vi "Register gRPC Methods.vi"(8 "error in (no error)":errorcluster, 11 "Template Server in":refnum<class "ctet_smu.lvclass">) -> (0 "error out":errorcluster, 3 "Template Server out":refnum<class "ctet_smu.lvclass">)   [LabVIEW 2019, in "ctet_smu.lvlib" / "ctet_smu.lvclass"]
uses:
  ctet_smu.lvclass
  typeDefs/Server Internal UEs.ctl
  typeDefs/Server Internal Message.ctl
  typeDefs/Server gRPC UEs.ctl
  gRPC lvSupport/Server API/typeDefs/gRPCId Cluster.ctl
  gRPC lvSupport/Server API/typeDefs/grpcId.ctl
  ctet_smu.lvclass/ctet_smu.ctl
  gRPC lvSupport/gprc-lvsupport.lvlib
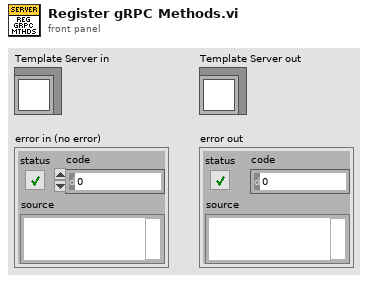
[diagram p1: front panel]
types:
  T1 = typedef "ctet_smu.lvlib/ctet_smu.lvclass/Server gRPC UEs.ctl" = cluster{"Invoke gRPC UE":refnum<user-event>, "Query gRPC UE":refnum<user-event>, "Register gRPC UE":refnum<user-event>, "OpenSMUSession gRPC UE":refnum<user-event>, "ConfigureSMU gRPC UE":refnum<user-event>, "EnableSMUOutput gRPC UE":refnum<user-event>, "DisableSMUOutput gRPC UE":refnum<user-event>, "PerformSMUCurrentMeasurement gRPC UE":refnum<user-event>, "CloseSMUSession gRPC UE":refnum<user-event>, "SelfCalibrateSMU gRPC UE":refnum<user-event>, "ResetSMU gRPC UE":refnum<user-event>, "GetSMULastExtCalInfo gRPC UE":refnum<user-event>, "GetSMULastSelfCalInfo gRPC UE":refnum<user-event>}
  T2 = typedef "ctet_smu.lvlib/ctet_smu.lvclass/Server Internal UEs.ctl" = cluster{"Invoke Internal UE":refnum<user-event>, "Query Internal UE":refnum<user-event>, "Register Internal UE":refnum<user-event>, "OpenSMUSession Internal UE":refnum<user-event>, "ConfigureSMU Internal UE":refnum<user-event>, "EnableSMUOutput Internal UE":refnum<user-event>, "DisableSMUOutput Internal UE":refnum<user-event>, "PerformSMUCurrentMeasurement Internal UE":refnum<user-event>, "CloseSMUSession Internal UE":refnum<user-event>, "SelfCalibrateSMU Internal UE":refnum<user-event>, "ResetSMU Internal UE":refnum<user-event>, "GetSMULastExtCalInfo Internal UE":refnum<user-event>, "GetSMULastSelfCalInfo Internal UE":refnum<user-event>}
  T3 = typedef "ctet_smu.lvlib/gprc-lvsupport.lvlib/grpcId.ctl" = u64
  T4 = typedef "ctet_smu.lvlib/ctet_smu.lvclass/Server Internal Message UE.ctl" = refnum<user-event>
  T5 = typedef "ctet_smu.lvlib/gprc-lvsupport.lvlib/gRPCId Cluster UE.ctl" = refnum<user-event>
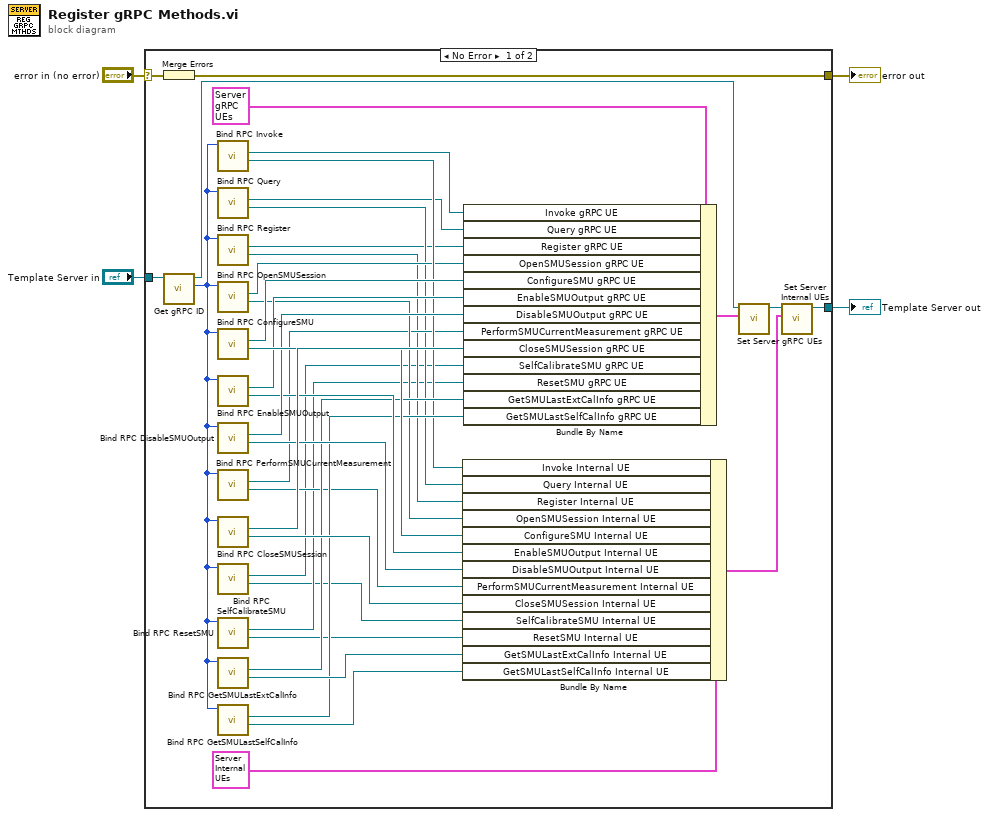
[diagram p0: block diagram]
diagram:
  n1 = case shown="No Error" "error in (no error)" {
    selector: "error in (no error)" -> [w32 w42]
    tunnel: "Template Server in" -> [w40 w43]
    tunnel: [w39 w42] -> w3
    tunnel: [w38 w43] -> w2
    frame No Error {
      n2 = Merge Errors(w32) -> (w39:errorcluster)
      n3 = call "Get gRPC ID.vi"("OOP Server in"=w40) -> ("gRPC ID"=w31:T3, "OOP Server out"=w41:refnum<class "ctet_smu.lvclass">)  [unwired: 9 in]
      n4 = call "Bind RPC Invoke.vi"("gRPCid server in"=w31) -> ("Invoke Internal UE"=w18:T4, "Invoke gRPC UE"=w17:T5)  [unwired: 7 in, 2 out]
      n5 = call "Bind RPC Query.vi"("gRPCid server in"=w31) -> ("Query Internal UE"=w12:T4, "Query gRPC UE"=w11:T5)  [unwired: 7 in, 2 out]
      n6 = call "Bind RPC Register.vi"("gRPCid server in"=w31) -> ("Register Internal UE"=w10:T4, "Register gRPC UE"=w9:T5)  [unwired: 7 in, 2 out]
      n7 = call "Bind RPC OpenSMUSession.vi"("gRPCid server in"=w31) -> ("OpenSMUSession Internal UE"=w16:T4, "OpenSMUSession gRPC UE"=w15:T5)  [unwired: 7 in, 2 out]
      n8 = call "Bind RPC ConfigureSMU.vi"("gRPCid server in"=w31) -> ("ConfigureSMU Internal UE"=w28:T4, "ConfigureSMU gRPC UE"=w27:T5)  [unwired: 7 in, 2 out]
      n9 = call "Bind RPC EnableSMUOutput.vi"("gRPCid server in"=w31) -> ("EnableSMUOutput Internal UE"=w24:T4, "EnableSMUOutput gRPC UE"=w23:T5)  [unwired: 7 in, 2 out]
      n10 = call "Bind RPC DisableSMUOutput.vi"("gRPCid server in"=w31) -> ("DisableSMUOutput Internal UE"=w26:T4, "DisableSMUOutput gRPC UE"=w25:T5)  [unwired: 7 in, 2 out]
      n11 = call "Bind RPC PerformSMUCurrentMeasurement.vi"("gRPCid server in"=w31) -> ("PerformSMUCurrentMeasurement Internal UE"=w14:T4, "PerformSMUCurrentMeasurement gRPC UE"=w13:T5)  [unwired: 7 in, 2 out]
      n12 = call "Bind RPC CloseSMUSession.vi"("gRPCid server in"=w31) -> ("CloseSMUSession Internal UE"=w30:T4, "CloseSMUSession gRPC UE"=w29:T5)  [unwired: 7 in, 2 out]
      n13 = call "Bind RPC SelfCalibrateSMU.vi"("gRPCid server in"=w31) -> ("SelfCalibrateSMU Internal UE"=w6:T4, "SelfCalibrateSMU gRPC UE"=w5:T5)  [unwired: 7 in, 2 out]
      n14 = call "Bind RPC ResetSMU.vi"("gRPCid server in"=w31) -> ("ResetSMU Internal UE"=w8:T4, "ResetSMU gRPC UE"=w7:T5)  [unwired: 7 in, 2 out]
      n15 = call "Bind RPC GetSMULastExtCalInfo.vi"("gRPCid server in"=w31) -> ("GetSMULastExtCalInfo Internal UE"=w22:T4, "GetSMULastExtCalInfo gRPC UE"=w21:T5)  [unwired: 7 in, 2 out]
      n16 = call "Bind RPC GetSMULastSelfCalInfo.vi"("gRPCid server in"=w31) -> ("GetSMULastSelfCalInfo Internal UE"=w20:T4, "GetSMULastSelfCalInfo gRPC UE"=w19:T5)  [unwired: 7 in, 2 out]
      n17 = Bundle By Name ("Bundle Internal UEs")(cluster=T2 {"Invoke Internal UE"=refnum, "Query Internal UE"=refnum, "Register Internal UE"=refnum, "OpenSMUSession Internal UE"=refnum, "ConfigureSMU Internal UE"=refnum, "EnableSMUOutput Internal UE"=refnum, "DisableSMUOutput Internal UE"=refnum, "PerformSMUCurrentMeasurement Internal UE"=refnum, "CloseSMUSession Internal UE"=refnum, "SelfCalibrateSMU Internal UE"=refnum, "ResetSMU Internal UE"=refnum, "GetSMULastExtCalInfo Internal UE"=refnum, "GetSMULastSelfCalInfo Internal UE"=refnum} ("Server Internal UEs"), "Invoke Internal UE"=w18, "Query Internal UE"=w12, "Register Internal UE"=w10, "OpenSMUSession Internal UE"=w16, "ConfigureSMU Internal UE"=w28, "EnableSMUOutput Internal UE"=w24, "DisableSMUOutput Internal UE"=w26, "PerformSMUCurrentMeasurement Internal UE"=w14, "CloseSMUSession Internal UE"=w30, "SelfCalibrateSMU Internal UE"=w6, "ResetSMU Internal UE"=w8, "GetSMULastExtCalInfo Internal UE"=w22, "GetSMULastSelfCalInfo Internal UE"=w20) -> (w37:T2)
      n18 = Bundle By Name ("Bundle gRPC UEs")(cluster=T1 {"Invoke gRPC UE"=refnum, "Query gRPC UE"=refnum, "Register gRPC UE"=refnum, "OpenSMUSession gRPC UE"=refnum, "ConfigureSMU gRPC UE"=refnum, "EnableSMUOutput gRPC UE"=refnum, "DisableSMUOutput gRPC UE"=refnum, "PerformSMUCurrentMeasurement gRPC UE"=refnum, "CloseSMUSession gRPC UE"=refnum, "SelfCalibrateSMU gRPC UE"=refnum, "ResetSMU gRPC UE"=refnum, "GetSMULastExtCalInfo gRPC UE"=refnum, "GetSMULastSelfCalInfo gRPC UE"=refnum} ("gRPC Server Method Events"), "Invoke gRPC UE"=w17, "Query gRPC UE"=w11, "Register gRPC UE"=w9, "OpenSMUSession gRPC UE"=w15, "ConfigureSMU gRPC UE"=w27, "EnableSMUOutput gRPC UE"=w23, "DisableSMUOutput gRPC UE"=w25, "PerformSMUCurrentMeasurement gRPC UE"=w13, "CloseSMUSession gRPC UE"=w29, "SelfCalibrateSMU gRPC UE"=w5, "ResetSMU gRPC UE"=w7, "GetSMULastExtCalInfo gRPC UE"=w21, "GetSMULastSelfCalInfo gRPC UE"=w19) -> (w34:T1)
      n19 = call "Set Server gRPC UEs.vi"("Server gRPC UEs"=w34, "OOP Server in"=w41) -> ("OOP Server out"=w35:refnum<class "ctet_smu.lvclass">)  [unwired: 9 in]
      n20 = call "Set Server Internal UEs.vi"("Server Internal UEs"=w37, "OOP Server in"=w35) -> ("OOP Server out"=w38:refnum<class "ctet_smu.lvclass">)  [unwired: 9 in]
    }
    frame Error {
    }
  }
  "error out" <- w3
  "Template Server out" <- w2
